vi "posi inicial-proceso 3.vi"() -> ()   [LabVIEW 2020]
panel:
  out "posi inicial-proceso 3":T1
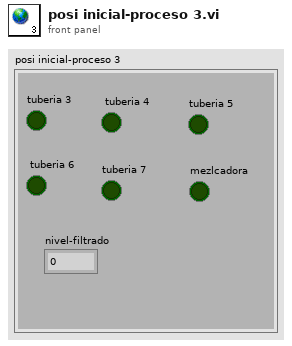
[diagram p1: front panel]
types:
  T1 = cluster{"tuberia 3":bool, " tuberia 4":bool, "tuberia 7":bool, "tuberia 5":bool, " tuberia 6":bool, "mezlcadora ":bool, "nivel-filtrado":dbl}
diagram:
